vi "Defer_FP_Updates.vi"(7 "Defer Panel Updates":bool, 8 "error in (no error)":errorcluster, 11 "lv_icon.vi in":refnum<vi>) -> (0 "error out":errorcluster, 3 "lv icon.vi out":refnum<vi>)   [LabVIEW 2021]
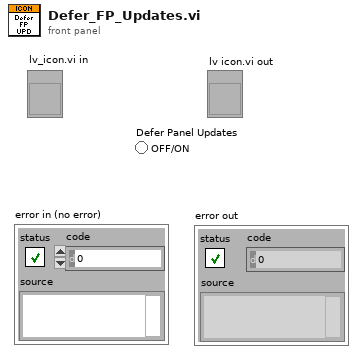
[diagram p1: front panel]
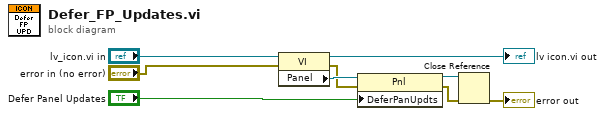
[diagram p0: block diagram]
diagram:
  n1 = property class="VI"(reference="lv_icon.vi in", error in="error in (no error)") -> (reference out=→"lv icon.vi out":refnum<vi>, error out=w7:errorcluster, "Panel"=w8:refnum<vi>)
  n2 = property class="Pnl"(reference=w8, error in=w7, "DeferPanUpdts"="Defer Panel Updates") -> (reference out=w5:refnum<vi>, error out=w6:errorcluster)
  n3 = Close Reference(reference=w5, error in (no error)=w6) -> (error out=→"error out":errorcluster)
